vi "GLOBAL_ACT Write_Data_Out.vi"() -> ()   [LabVIEW 2016, in "Compressor.lvlib"]
uses:
  Compressor.lvlib
  Shared/TypeDef/Cluster_Compressor.ctl
panel:
  out "Compressor Cluster":T1
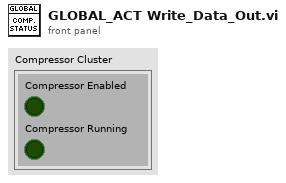
[diagram p1: front panel]
types:
  T1 = typedef "Cluster_Compressor.ctl" = cluster{"Compressor Running":bool, "Compressor Enabled":bool}
diagram:
